vi "Save Display Settings2File.vi"(0 "Display State In":T2 {"ROI"."Contours"."Type" items=["No Selection", "Point", "Line", "Rectangle", "Oval", "Polygon", "Freehand Region", "Annulus", "Unused2", "Unused3", "Broken Line", "Freehand Line", "Rotated Rectangle"]}, 9 "Container State":T7, 11 "error in (no error)":errorcluster) -> (4 "Display State Out":T2 {"ROI"."Contours"."Type" items=["No Selection", "Point", "Line", "Rectangle", "Oval", "Polygon", "Freehand Region", "Annulus", "Unused2", "Unused3", "Broken Line", "Freehand Line", "Rotated Rectangle"]}, 6 "file path out":path, 15 "error out":errorcluster)   [LabVIEW 2009, in "POLARIS IMAQ Display.xctl"]
doc: "use this method via invoke node in Your application to save XControl settings in the configuration file.\n\nLast update:\n\n\nauthor: Alexander Kessler, Helmholtz-Institut-Jena \nmaintainer: Alexander Kessler: alexander.kessler@uni-jena.de\n\n\n\nLicense Agreement for this software:\n\nCopyright (C)\nHelmholtz-Institut-Jena\nFröbelstieg 3\n07743 Jena\nGermany\n\nThis program is free software; you can redistribute it and/or modify it under the terms of the GNU General Public License as published by the Free Software Foundation; either version 2 of the license, or (at your option) any later version.\n\nThis program is distributed in the hope that it will be useful, but WITHOUT ANY WARRANTY; without even the implied warranty of MERCHANTABILITY or FITNESS FOR A PARTICULAR PURPOSE. See the GNU General License for more details (http://www.gnu.org)."
uses:
  POLARIS IMAQ Display.xctl
  <vilib>/_xctls/Container State.ctl
  State.ctl
  IMAQdx Cam/IMAQdx Cam.lvclass
  Properties/ImageSource.ctl
  <vilib>/vision/Image Controls.llb/IMAQ Image.ctl
  DisplaySettings.ctl
  Named ROI.ctl
  Analyze Classes/Analyze BaseClass/Analyze BaseClass.lvclass
  <vilib>/_xctls/XControlSupport.lvlib
panel:
  out "Image":T1(plugin-control)
  # "Add Controls & Indicators that form the parameters of the method here. Hook them to the connector pane. Do not delete the controls & indicators that are already hooked to the connector pane.\n \nTo setup the parameters  for this method, right click on this item in the Project Tree & select \"Configure Method...\"."
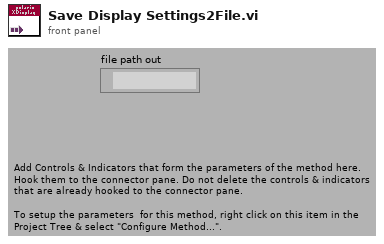
[diagram p1: front panel]
types:
  T1 = typedef "IMAQ Image.ctl" = refnum<image>
  T2 = typedef "POLARIS IMAQ Display.xctl/State.ctl" = cluster{"ImageSource":T3, "IMAQdx Cam":refnum<class "IMAQdx Cam.lvclass">, "WorkDir":path, "Image Name Prefix":string, "ROI":T4, "BG Image":T1, "Display Image":T1, "Display settings":T5, "Mask image":T1, "ConfigDir":path, "Display ref":refnum<vi>, "Saved ROIs":T6[], "Selected ROI":string, "Analyze Objects":refnum<class "Analyze BaseClass.lvclass">[], "Analysis Params":variant, "Analysis Results":variant, "Overlays?":bool[]}
  T3 = typedef "POLARIS IMAQ Display.xctl/ImageSource.ctl" = enum16{"Camera", "File"}
  T4 = typedef "ROI Descriptor" = cluster{"Global Rectangle":i32[], "Contours":cluster{"ID":enum32{"External", "Internal"}, "Type":u32, "Coordinates":i32[]}[]}
  T5 = typedef "POLARIS IMAQ Display.xctl/DisplaySettings.ctl" = cluster{"Min. Thresh.":sgl, "X":dbl, "Y":dbl, "ShowLineout":bool, "ScaleParts":i32, "ShowLegende":bool, "Target Cross":bool, "Centroid Cross":bool, "Target color":u32, "Centroid color":u32, "calibr. mm/px":sgl}
  T6 = typedef "POLARIS IMAQ Display.xctl/Named ROI.ctl" = cluster{"ROI":cluster{"Global Rectangle":i32[], "Contours":cluster{"Contour Type":u32, "ROI Type":u32, "Points":i32[]}[]}, "Name":string}
  T7 = typedef "XControlSupport.lvlib/Container State.ctl" = cluster{"Indicator?":bool, "Run Mode?":bool, " Refnum":refnum<vi>}
  T8 = cluster{"Global Rectangle":i32[], "Contours":cluster{"Contour Type":u32, "ROI Type":u32, "Points":i32[]}[]}
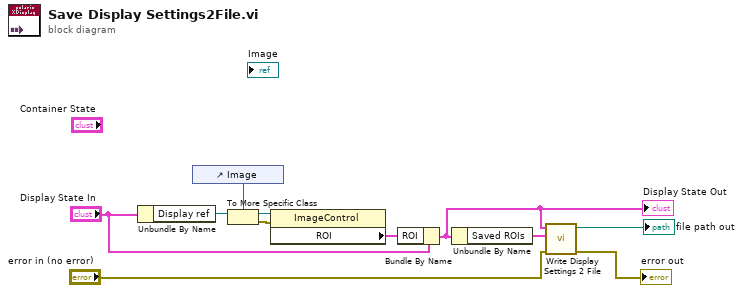
[diagram p0: block diagram]
diagram:
  n1 = Unbundle By Name("Display State In") -> ("Display ref"=w5:refnum<vi>)
  n2 = control-ref of="Image"() -> (w6:refnum<vi>)
  n3 = To More Specific Class(target class=w6, reference=w5) -> (specific class reference=w7:refnum<vi>, error out=w8:errorcluster)  [unwired: 1 in]
  n4 = property class="ImageControl"(reference=w7, error in=w8) -> ("ROI"=w2:T8)  [unwired: 2 out]
  n5 = Bundle By Name(cluster="Display State In", "ROI"=w2) -> (w3:T2)
  "Display State Out" <- w3
  n6 = Unbundle By Name(w3) -> ("Saved ROIs"=w9:T6[])
  n7 = call "Write Display Settings 2 File.vi"("error in"="error in (no error)", "Saved ROIs"=w9, "State"=w3) -> ("error out"=→"error out":errorcluster, "file path out"=→"file path out":path)  [unwired: 7 in]
